vi "Autonomous Independent Backup 4th feb.vi"() -> ()   [LabVIEW 2016]
uses:
  <vilib>/Rock Robotics/WPI/Utilities/WPI_GetSetVariantRefNum.vi
  <vilib>/Rock Robotics/Network Tables/NT Read String.vi
  <vilib>/Rock Robotics/Network Tables/NT Write Numeric Array.vi
  <vilib>/Rock Robotics/WPI/RobotDrive/WPI_RobotDriveArcadeDrive_Standard(NoSaturation).vi
  <vilib>/Rock Robotics/SystemInterfaces/DIO/FPGA_DIOChannel.ctl
  <vilib>/Rock Robotics/WPI/Counter/WPI_CounterDigitalInputToDigitalSource.vi
panel:
  out "Current Movement, for debugging 2":T1 {"Y Joystick Value" scale=1.0..-1.0; "X Joystick Value" scale=-1.0..1.0}
  in  "Array of robot movements 2":T2(array[cluster])=[{"X Joystick Value"=0.39393939393939403, "Y Joystick Value"=0.0, "Delay (sec)"=1.0, "Movement Name"="turn"}, {"X Joystick Value"=-0.3737373737373737, "Y Joystick Value"=0.0, "Delay (sec)"=1.0, "Movement Name"="turn back"}] {"Y Joystick Value" scale=1.0..-1.0; "X Joystick Value" scale=-1.0..1.0}
  out "Encoder Direction 3":string
  out "Encoder Distance 3":dbl
  out "Switch Pressed":bool
  out "Motor Values":dbl[](array[numeric])
  out "Encoder Direction":string
  out "Encoder Distance":dbl
  out "Encoder Direction 2":string
  out "Encoder Distance 2":dbl
  out "Current Movement, for debugging":T1 {"Y Joystick Value" scale=1.0..-1.0; "X Joystick Value" scale=-1.0..1.0}
  in  "Array of robot movements":T2(array[cluster])=[{"X Joystick Value"=0.39393939393939403, "Y Joystick Value"=0.0, "Delay (sec)"=1.0, "Movement Name"="turn"}, {"X Joystick Value"=-0.3737373737373737, "Y Joystick Value"=0.0, "Delay (sec)"=1.0, "Movement Name"="turn back"}] {"Y Joystick Value" scale=1.0..-1.0; "X Joystick Value" scale=-1.0..1.0}
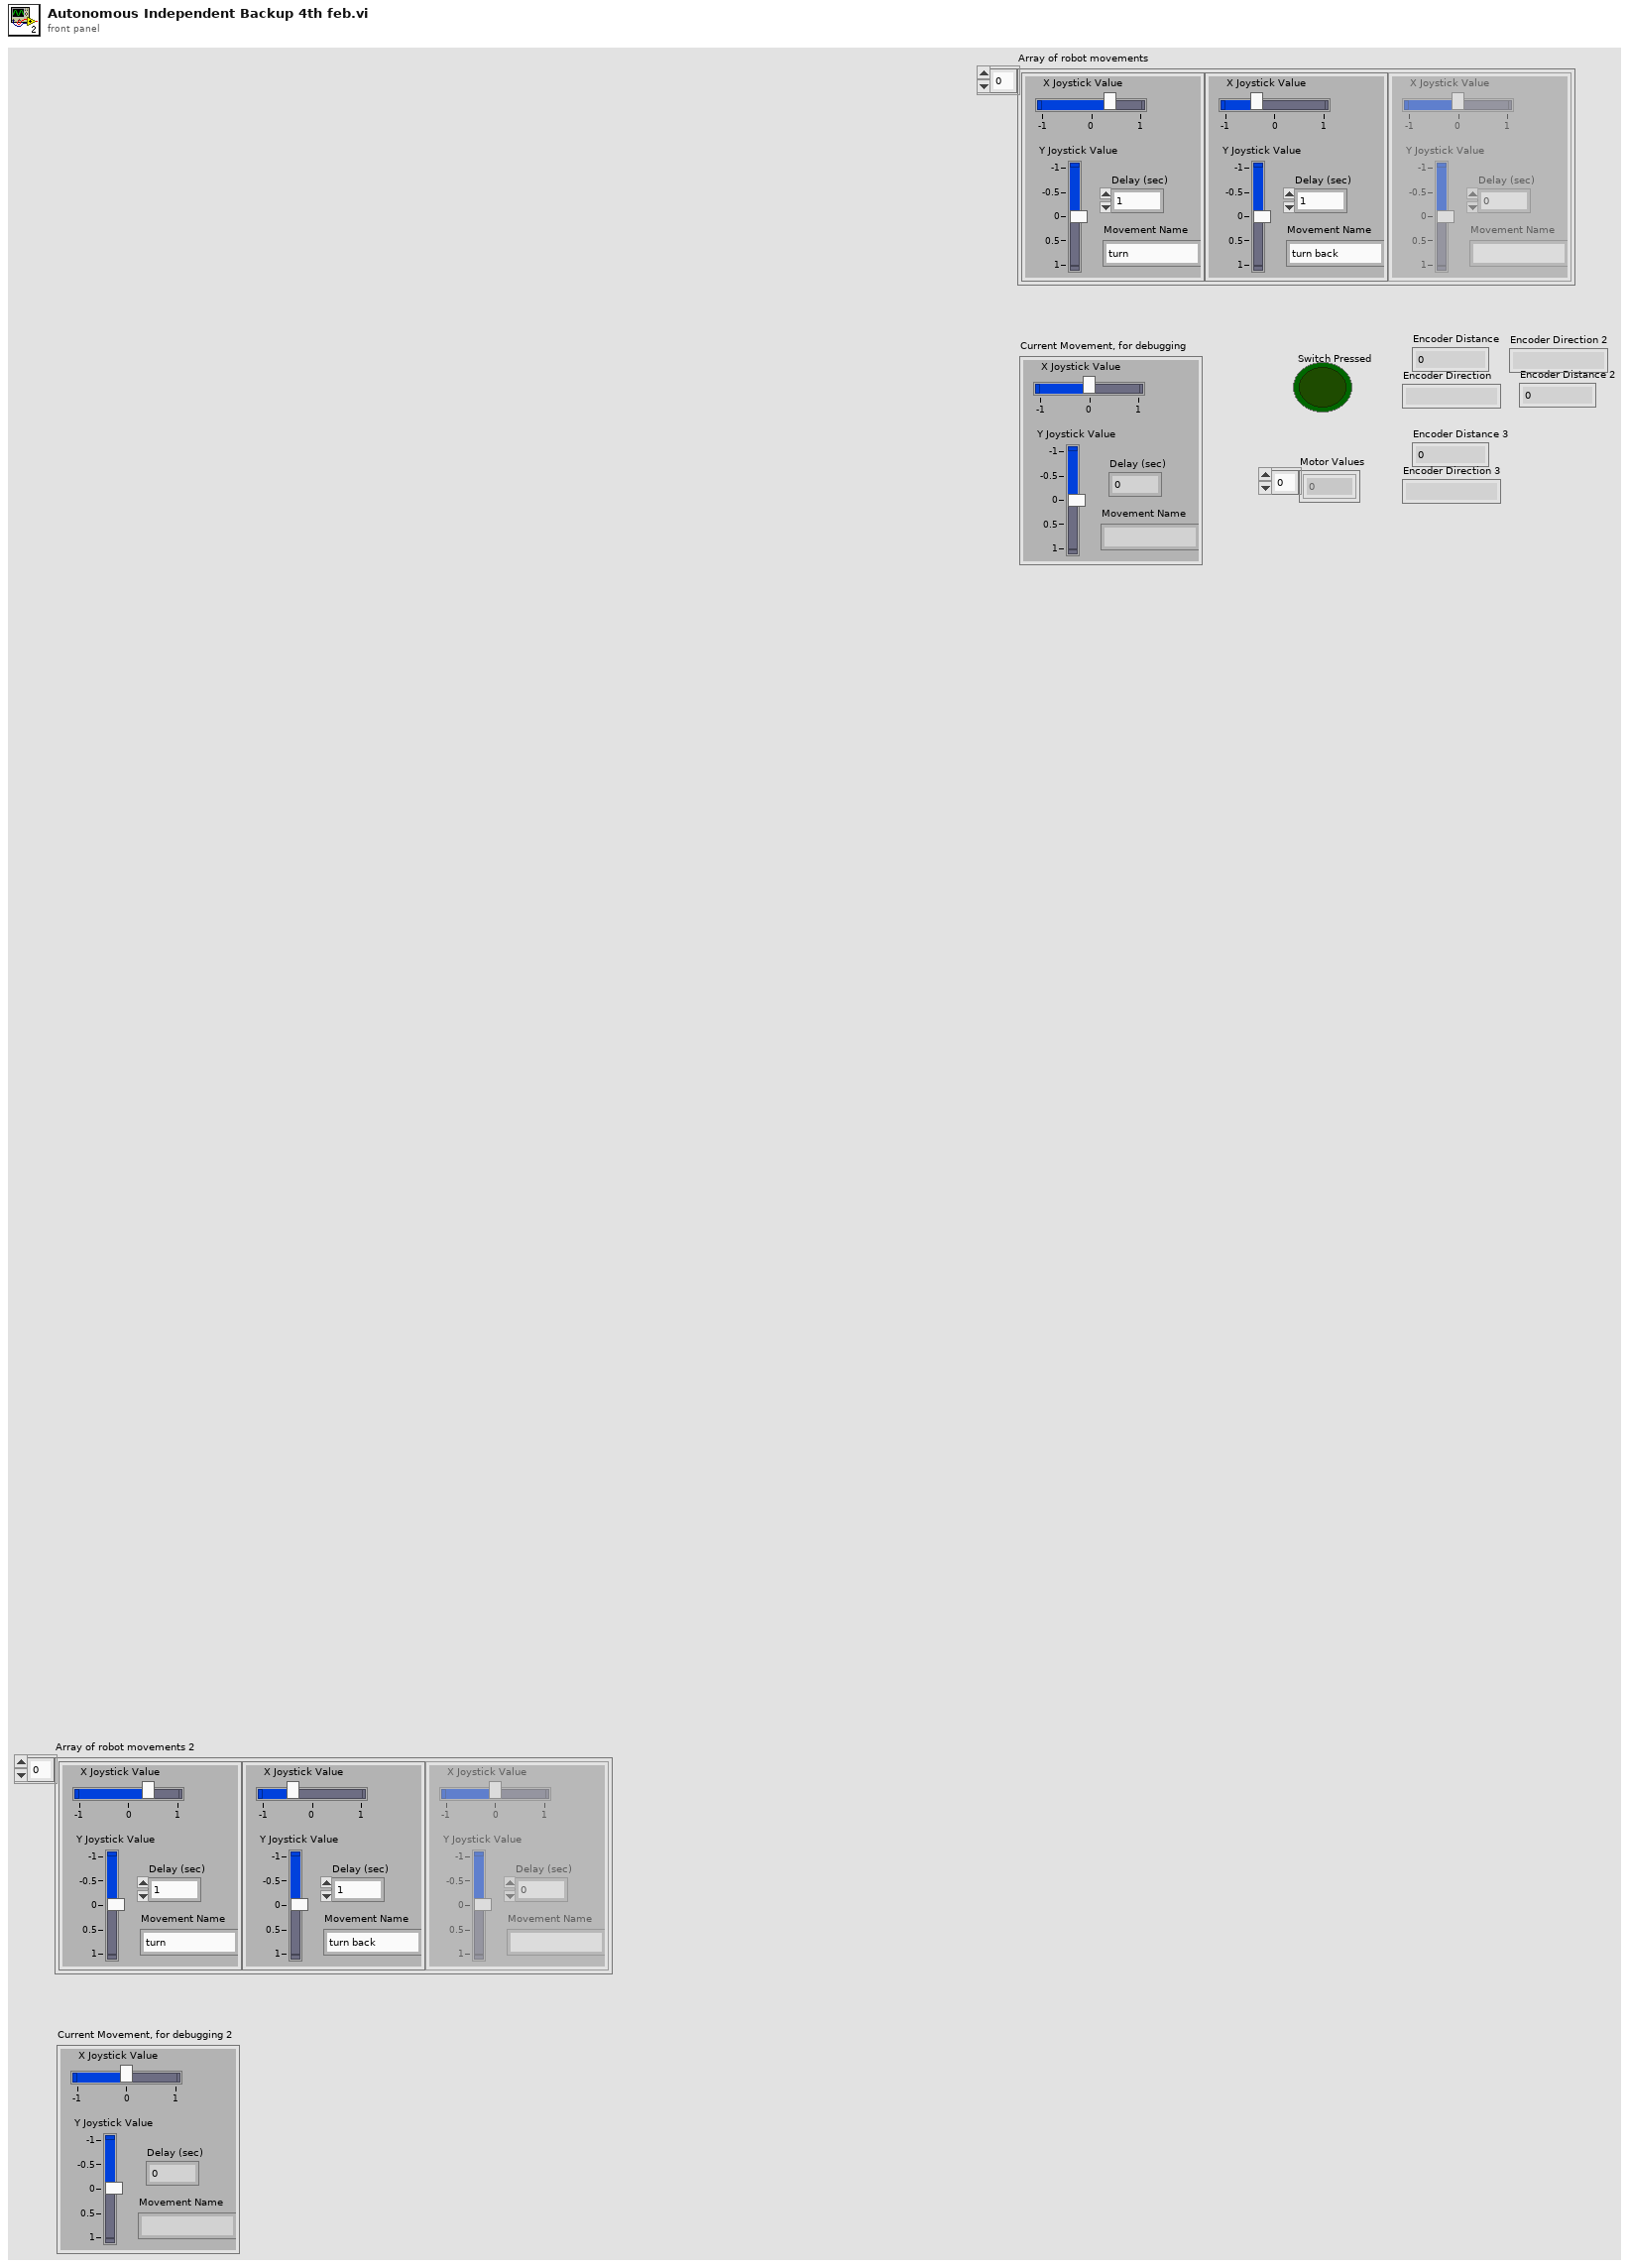
[diagram p1: front panel]
types:
  T1 = cluster{"X Joystick Value":dbl, "Y Joystick Value":dbl, "Delay (sec)":dbl, "Movement Name":string}
  T2 = cluster{"X Joystick Value":dbl, "Y Joystick Value":dbl, "Delay (sec)":dbl, "Movement Name":string}[]
  T3 = typedef "WPI_DriverStationPositionInfo.ctl" = enum16{"1", "2", "3"}
  T4 = typedef "WPI_RobotDriveDevRef.ctl" = cluster{"DevStatus":errorcluster, "Motors[]":T5[], "Square Inputs":bool, "Max Output":dbl}
  T5 = typedef "WPI_MotorControlDeviceRef.ctl" = cluster{"DeviceStatus":errorcluster, "Type":T6, "PWM":cluster{"PWM Channel":T7, "DeadBand":T8}, "CAN":cluster{"Device Number":u8, "SetOutput VI Ref":variant, "GetOutput VI Ref":variant, "Enable VI Ref":variant, "Disable VI Ref":variant, "Data":variant}, "Invert":bool}
  T6 = typedef "WPI_MotorControlType.ctl" = enum16{"PWM", "CAN"}
  T7 = typedef "FPGA_DIOPWMChannel.ctl" = enum8{"PWM 0", "PWM 1", "PWM 2", "PWM 3", "PWM 4", "PWM 5", "PWM 6", "PWM 7", "PWM 8", "PWM 9", "PWM MXP 0", "PWM MXP 1", "PWM MXP 2", "PWM MXP 3", "PWM MXP 4", "PWM MXP 5", "PWM MXP 6", "PWM MXP 7", "PWM MXP 8", "PWM MXP 9", "Invalid"}
  T8 = typedef "WPI_PWMDeadband.ctl" = cluster{"Name":string, "maxPositivePwm":i32, "minPositivePwm":i32, "centerPwm":i32, "maxNegativePwm":i32, "minNegativePwm":i32, "angularRange":u16}
  T9 = typedef "FPGA_DIOChannel.ctl" = enum8{"DIO 0", "DIO 1", "DIO 2", "DIO 3", "DIO 4", "DIO 5", "DIO 6", "DIO 7", "DIO 8", "DIO 9", "DIO MXP 0", "DIO MXP 1", "DIO MXP 2", "DIO MXP 3", "DIO MXP 4", "DIO MXP 5", "DIO MXP 6", "DIO MXP 7", "DIO MXP 8", "DIO MXP 9", "DIO MXP 10", "DIO MXP 11", "DIO MXP 12", "DIO MXP 13", "DIO MXP 14", "DIO MXP 15", "SPI Port CS1", "SPI Port CS2", "SPI Port CS3", "SPI Port MISO", "SPI Port MOSI", "Invalid"}
  T10 = typedef "WPI_DigitalInputDevRef.ctl" = cluster{"DevStatus":errorcluster, "DIO Channel":T9}
  T11 = typedef "FPGA_CounterEncoderSourceConvertionLVSourceType.ctl" = cluster{"DevStatus":errorcluster, "AnalogTriggerMode?":bool, "DigitalMode":cluster{"DIO Channel":T12}, "AnalogTriggerMode":cluster{"AnalogTriggerIndex":T13, "OutputType":T14}}
  T12 = typedef "FPGA_DIODigitalSourceChannel.ctl" = enum8{"DIO 0", "DIO 1", "DIO 2", "DIO 3", "DIO 4", "DIO 5", "DIO 6", "DIO 7", "DIO 8", "DIO 9", "DIO MXP 0", "DIO MXP 1", "DIO MXP 2", "DIO MXP 3", "DIO MXP 4", "DIO MXP 5", "DIO MXP 6", "DIO MXP 7", "DIO MXP 8", "DIO MXP 9", "DIO MXP 10", "DIO MXP 11", "DIO MXP 12", "DIO MXP 13", "DIO MXP 14", "DIO MXP 15", "Disabled"}
  T13 = typedef "FPGA_AnalogTriggerIndex.ctl" = enum8{"Trig 0", "Trig 1", "Trig 2", "Trig 3", "Trig 4", "Trig 5", "Trig 6", "Trig 7", "Invalid"}
  T14 = typedef "FPGA_AnalogTriggerOutType.ctl" = enum16{"InWindow", "TriggerState", "Rising", "Falling"}
  T15 = typedef "WPI_EncoderDevRef.ctl" = cluster{"DevStatus":errorcluster, "EncoderIndex":T16, "CounterIndex":T17, "DistancePerCount":dbl, "Decoding Type":T18}
  T16 = typedef "FPGA_EncoderIdx.ctl" = enum8{"Enc 0", "Enc 1", "Enc 2", "Enc 3", "Enc 4", "Enc 5", "Enc 6", "Enc 7", "Invalid"}
  T17 = typedef "FPGA_CounterCtrSystemIndex.ctl" = enum8{"Ctr 0", "Ctr 1", "Ctr 2", "Ctr 3", "Ctr 4", "Ctr 5", "Ctr 6", "Ctr 7", "Invalid"}
  T18 = typedef "WPI_EncoderType.ctl" = enum16{"1x", "2x", "4x"}
  T19 = typedef "WPI_JoystickDevRef.ctl" = cluster{"Device":T20}
  T20 = typedef "WPI_JoystickDeviceEnum.ctl" = enum16{"USB 0", "USB 1", "USB 2", "USB 3", "USB 4", "USB 5"}
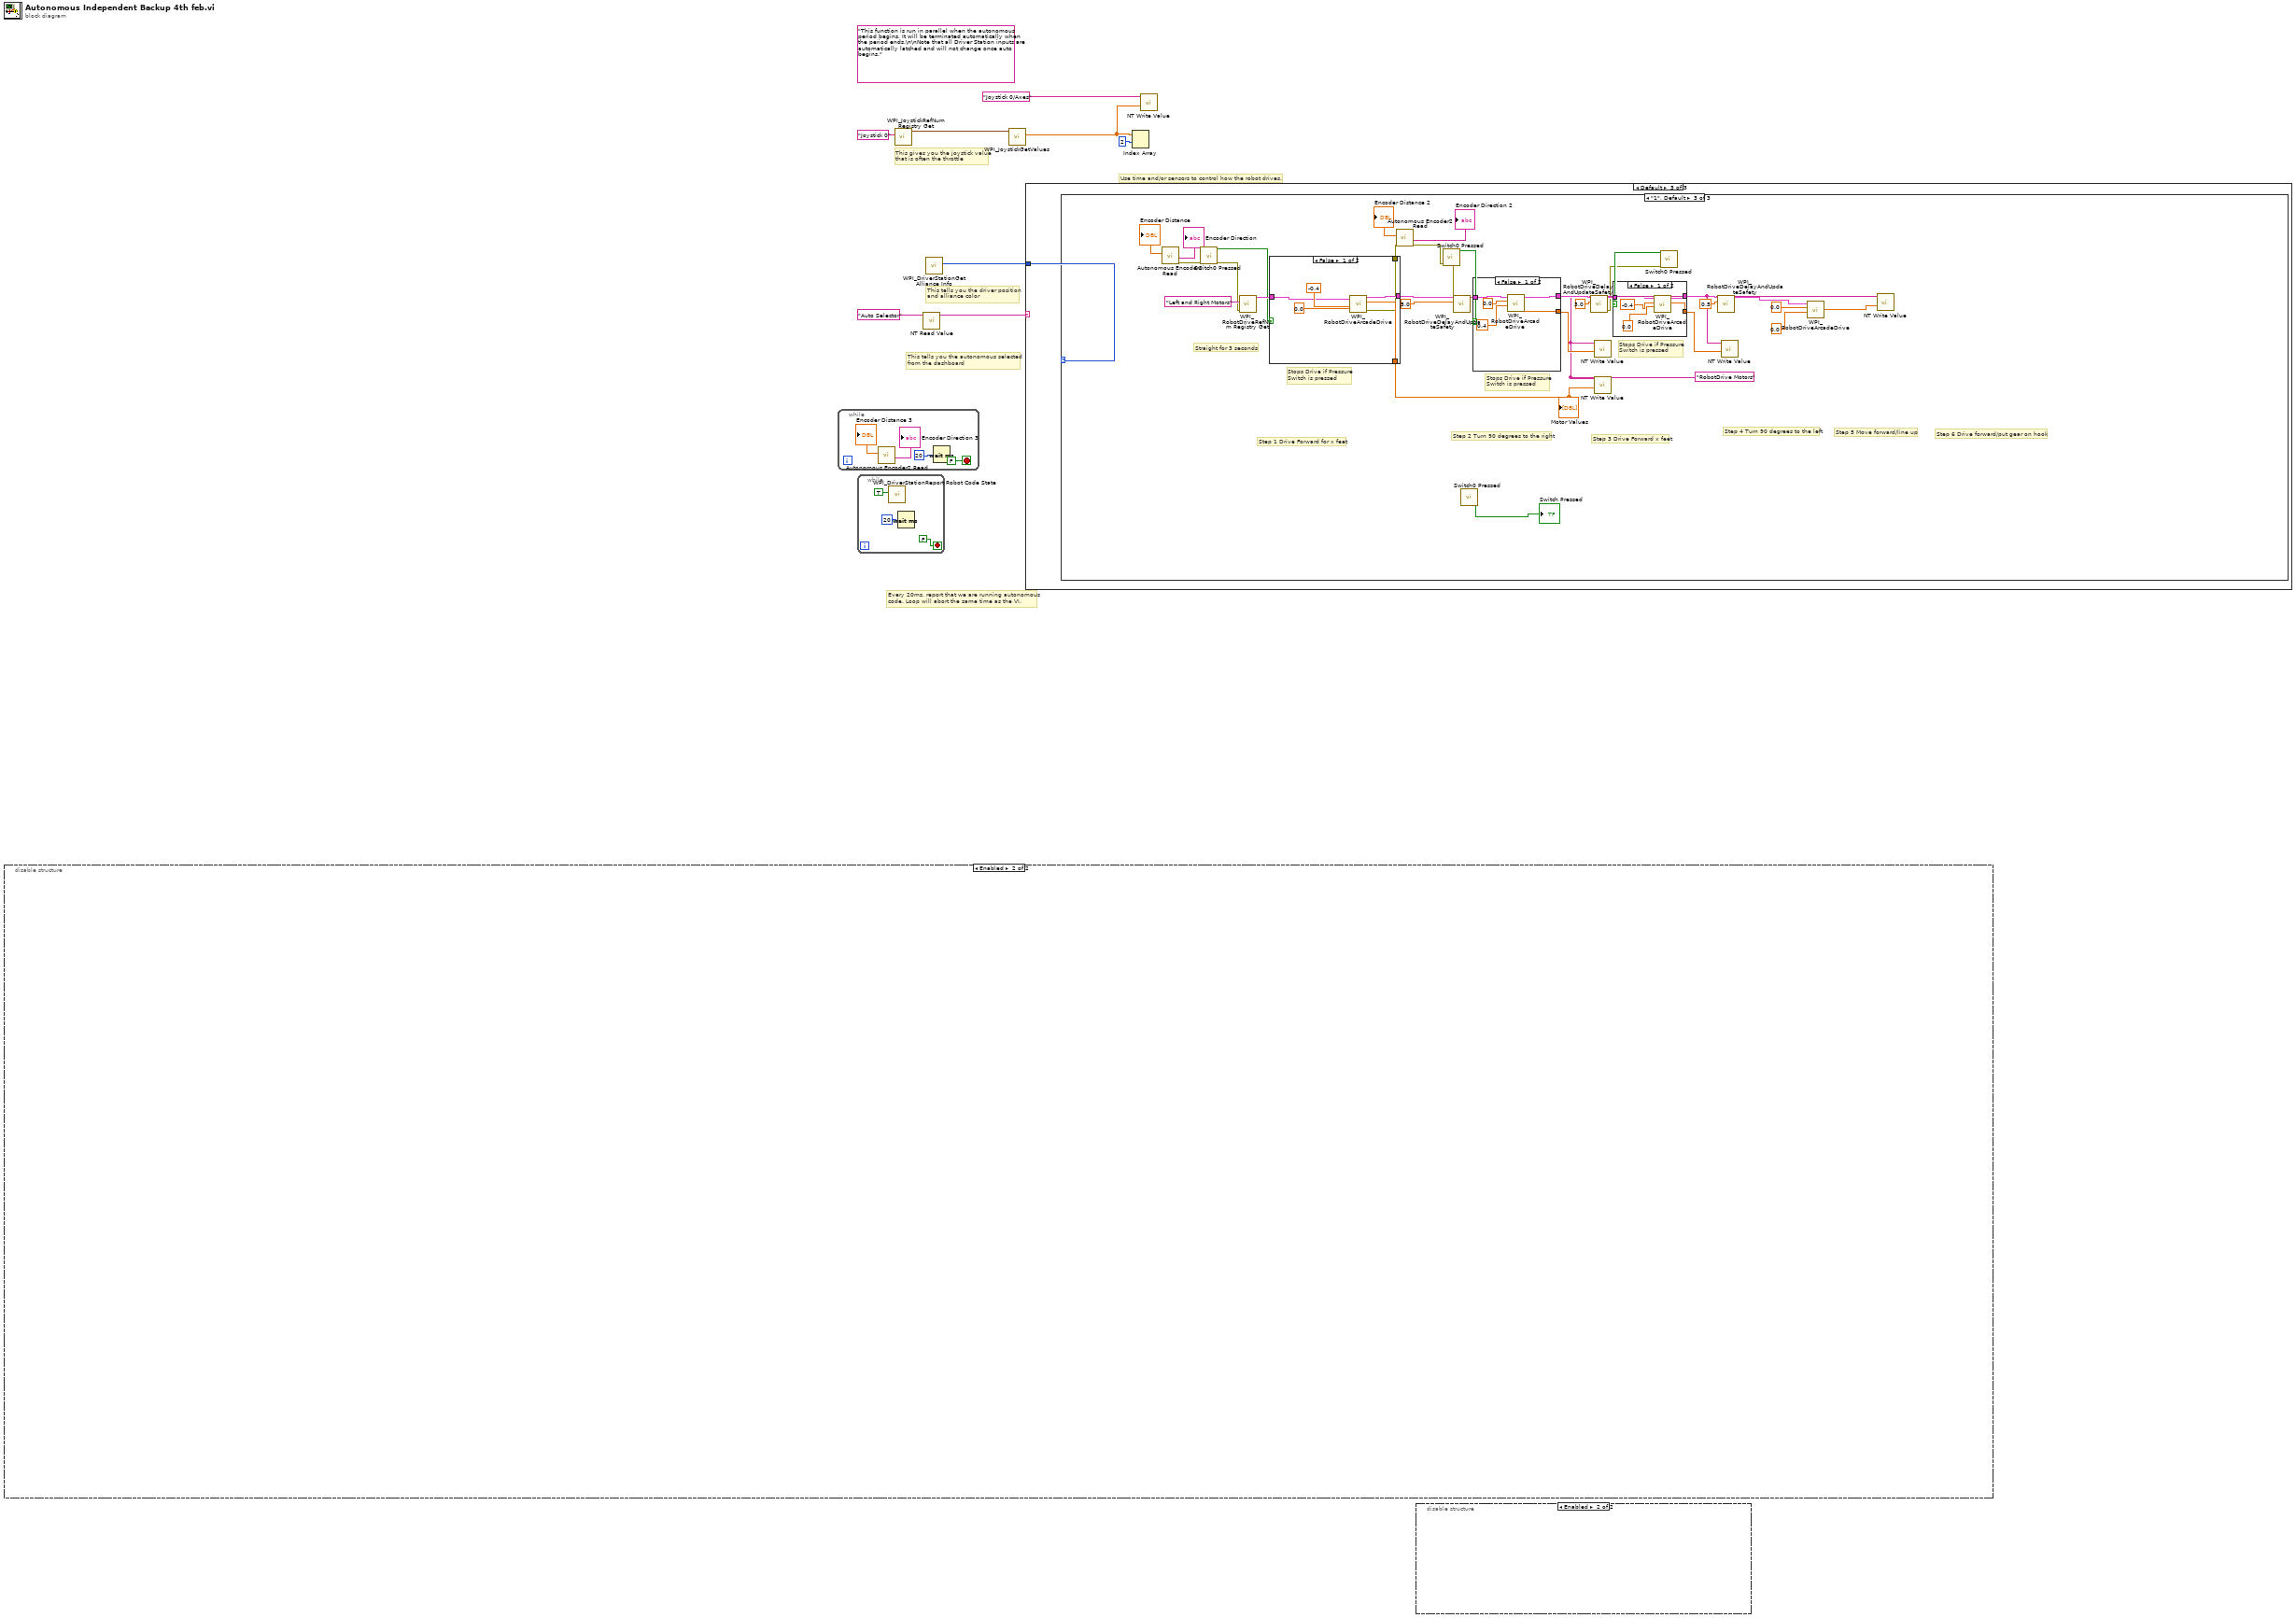
[diagram p0: block diagram]
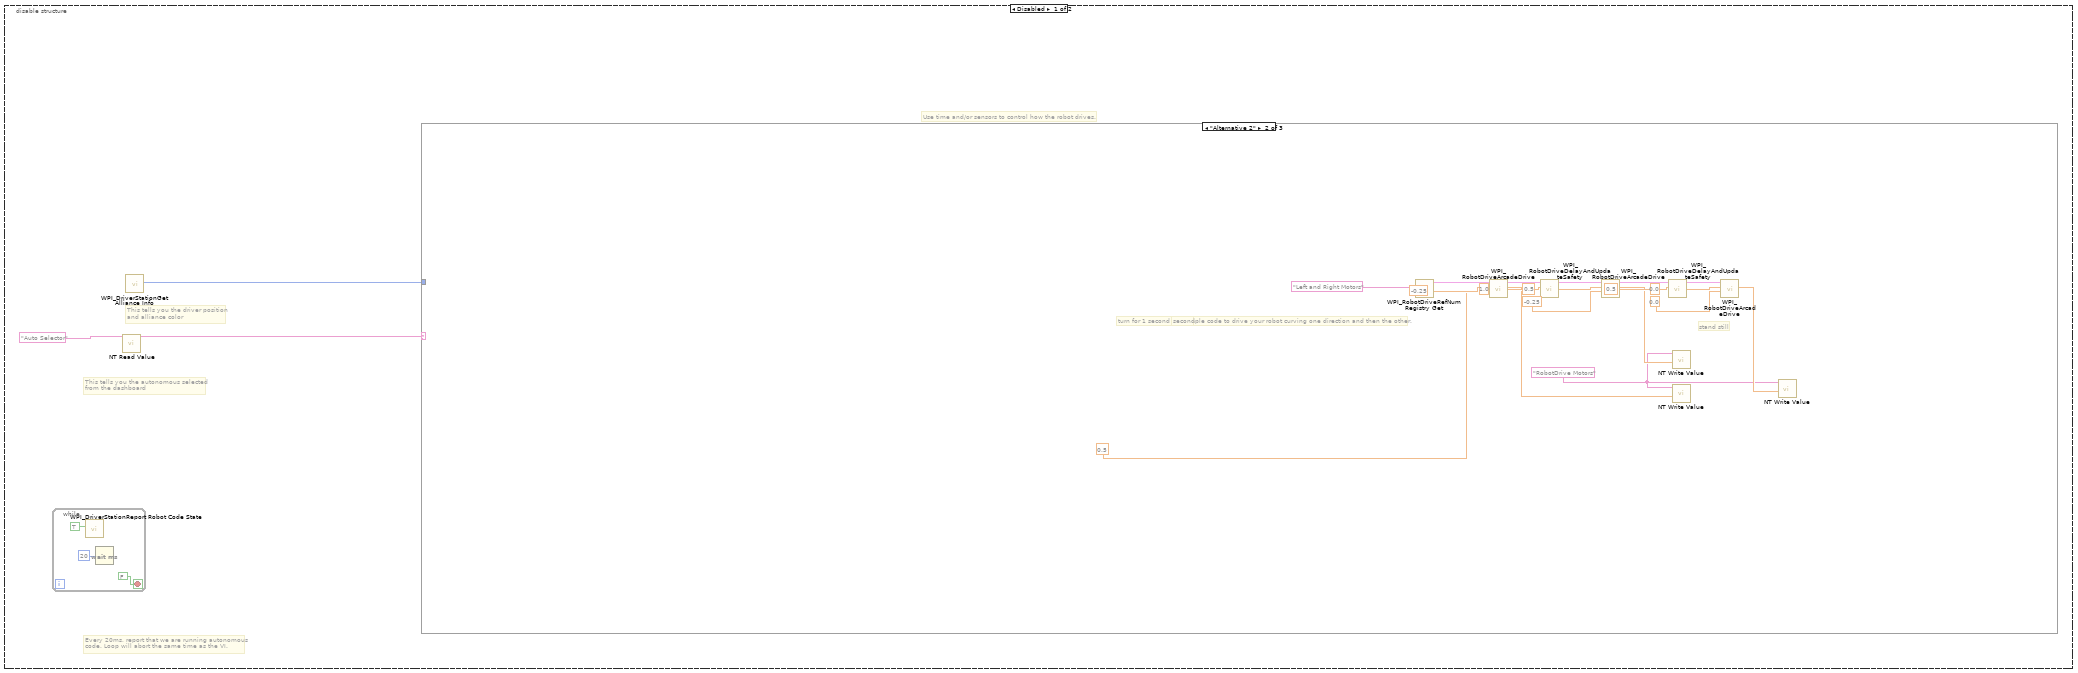
[diagram p2: hidden frame]
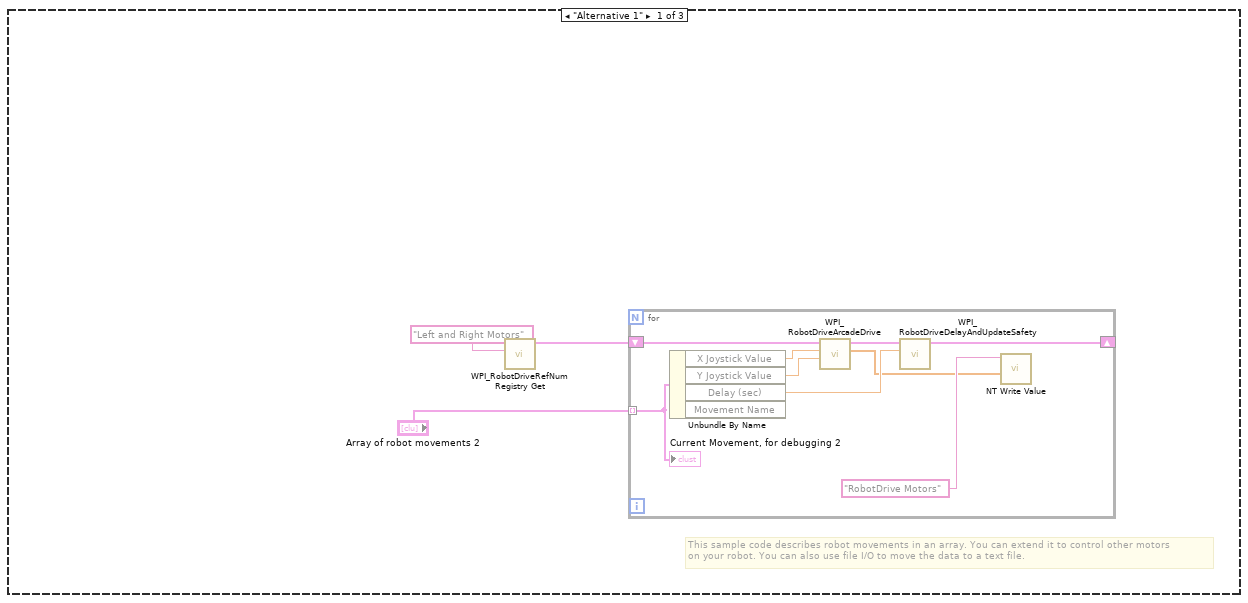
[diagram p3: hidden frame]
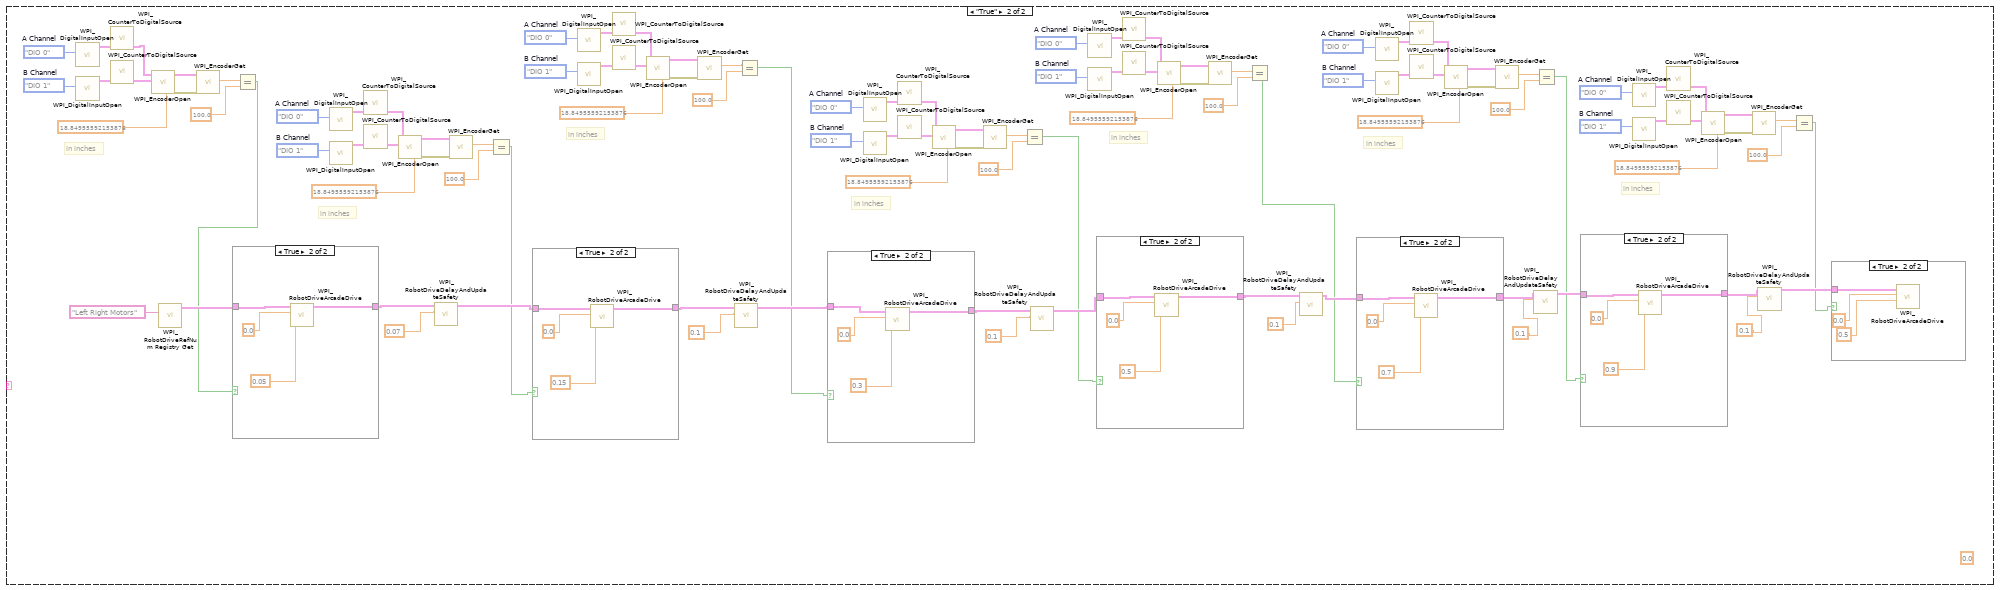
[diagram p5: hidden frame]
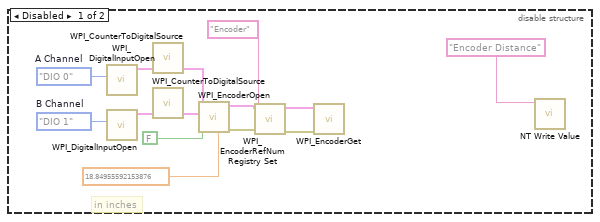
[diagram p13: hidden frame]
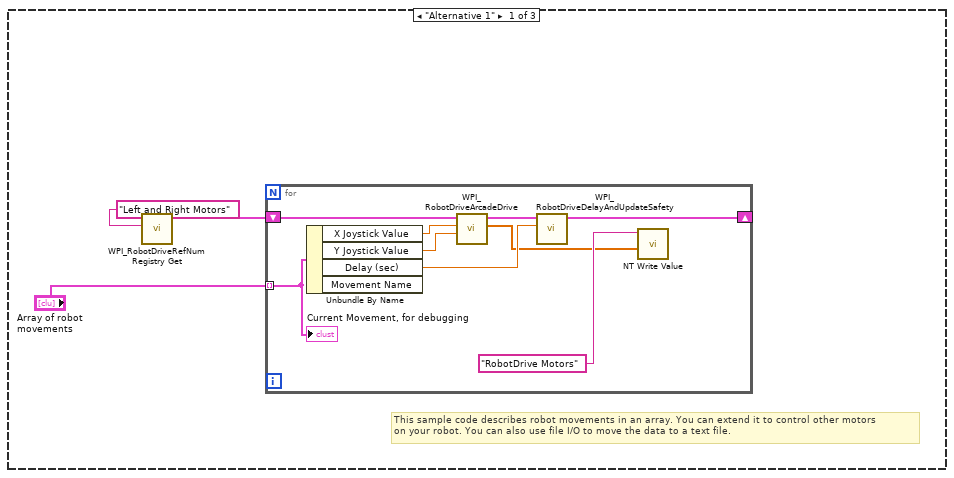
[diagram p14: hidden frame]
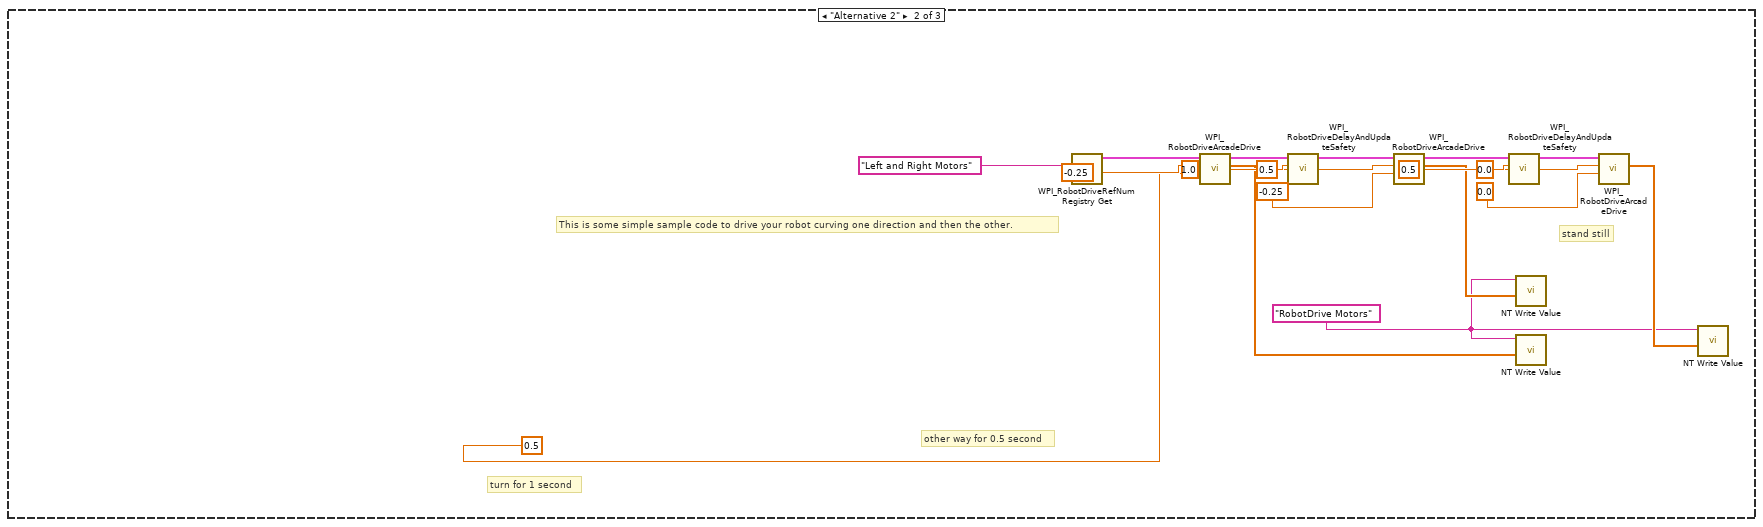
[diagram p15: hidden frame]
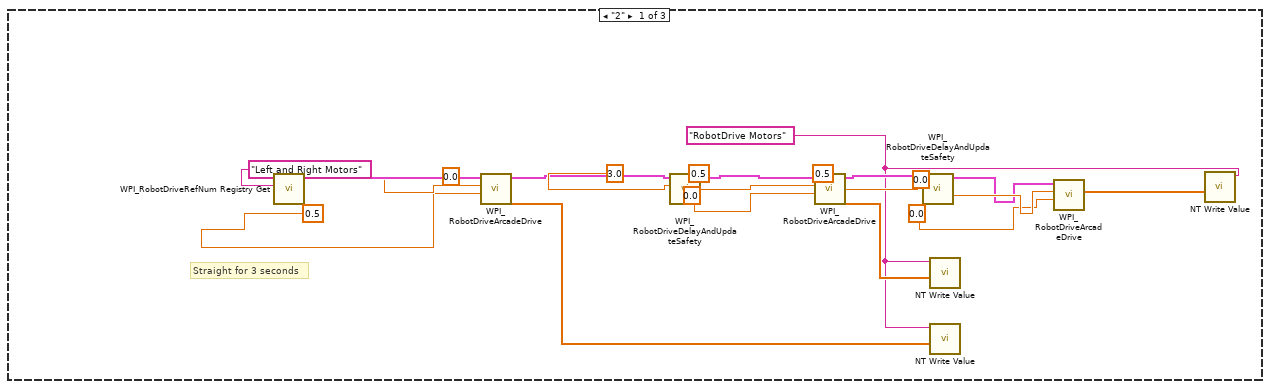
[diagram p16: hidden frame]
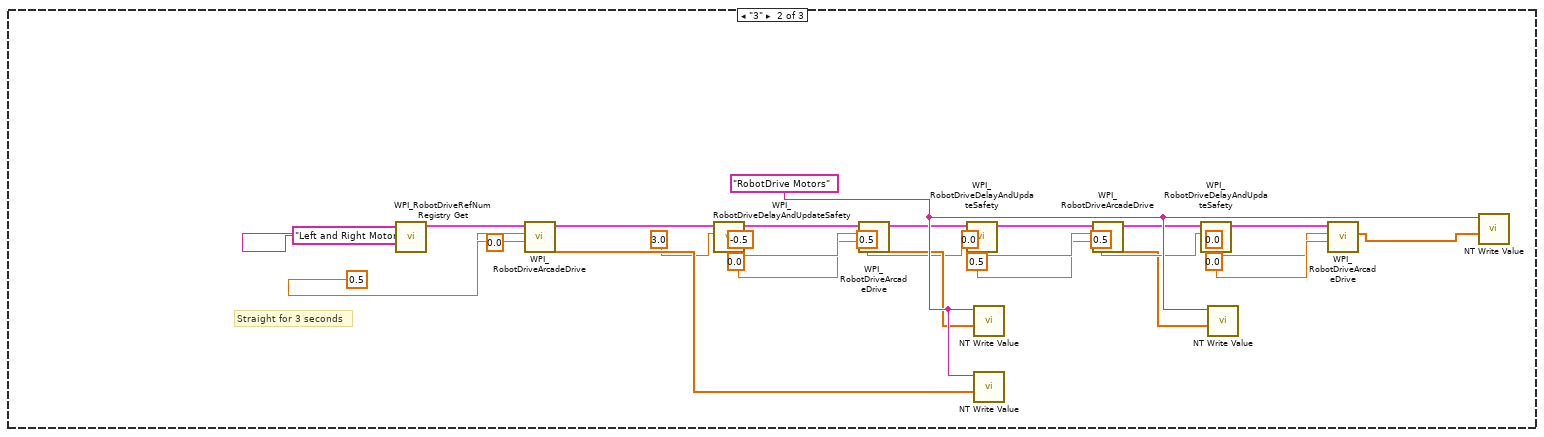
[diagram p17: hidden frame]
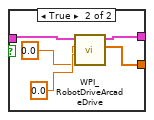
[diagram p18: hidden frame]
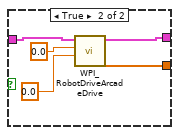
[diagram p19: hidden frame]
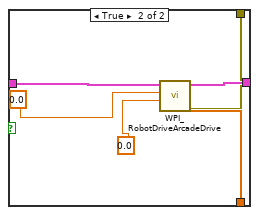
[diagram p20: hidden frame]
diagram:
  (unwired) "This function is run in parallel when the autonomous period begins. It will be terminated automatically when the period ends.\n\nNote that all Driver Station inputs are automatically latched and will not change once auto begins."
  # "This tells you the autonomous selected\nfrom the dashboard"
  # "Every 20ms, report that we are running autonomous\ncode. Loop will abort the same time as the VI."
  # "This gives you the joystick value\nthat is often the throttle"
  # "Use time and/or sensors to control how the robot drives."
  # "This tells you the driver position\nand alliance color"
  n1 = disable-structure shown="Enabled" {
    frame Disabled {
      # "This tells you the autonomous selected\nfrom the dashboard"
      # "Every 20ms, report that we are running autonomous\ncode. Loop will abort the same time as the VI."
      # "Use time and/or sensors to control how the robot drives."
      # "This tells you the driver position\nand alliance color"
      n2 = while {
        stop <- FALSE stop-if-true
        n3 = call <vilib>:"WPI_DriverStationReport Robot Code State.vi"("Autonomous"=TRUE) -> ()  [unwired: 10 in, 1 out]
        n4 = Wait (ms)(milliseconds to wait=u32 20) -> ()  [unwired: 1 out]
      }
      n5 = call-poly <vilib>:"NT Read Value.vi"("Name"="Auto Selector") -> ("String"=w11:string)  [unwired: 9 in, 1 out]
      n6 = call <vilib>:"WPI_DriverStationGet Alliance Info.vi"() -> ("Position"=w10:T3)  [unwired: 11 out]
      n7 = case shown="\"Alternative 2\"" w11 {
        selector: w11 -> [_ _ w42]
        tunnel: w10 -> [_ _ _]
        frame "Alternative 1" {
          # "This sample code describes robot movements in an array. You can extend it to control other motors\non your robot. You can also use file I/O to move the data to a text file."
          n8 = call <vilib>:"WPI_RobotDriveRefNum Registry Get.vi"("refnum name"="Left and Right Motors") -> ("RobotDriveDevRef"=w13:T4)  [unwired: 1 in, 9 out]
          n9 = for {
            shift-right: [w21] -> _
            shift-left: w13 -> [w22]
            tunnel: "Array of robot movements 2" -> [w17] mode=indexing
            n10 = Unbundle By Name(w17) -> ("X Joystick Value"=w20:dbl, "Y Joystick Value"=w19:dbl, "Delay (sec)"=w18:dbl)  [unwired: 1 out]
            n11 = call-poly <vilib>:"WPI_RobotDriveArcadeDrive.vi"("Y axis value"=w19, "X axis value"=w20, "RobotDriveDevRef"=w22) -> ("Motor Values"=w15:dbl[], "RobotDriveDevRef"=w23:T4)  [unwired: 1 in, 6 out]
            n12 = call <vilib>:"WPI_RobotDriveDelayAndUpdateSafety.vi"("Delay (s)"=w18, "RobotDriveDevRef"=w23) -> ("RobotDriveDevRef 2"=w21:T4)  [unwired: 8 in, 1 out]
            n13 = call-poly <vilib>:"NT Write Value.vi"("Numeric Array"=w15, "Name"="RobotDrive Motors") -> ()  [unwired: 9 in, 1 out]
            "Current Movement, for debugging 2" <- w17
          }
        }
        frame "Alternative 2" {
          w25 = "RobotDrive Motors" ("Name")
          # "This is some simple sample code to drive your robot curving one direction and then the other."
          # "stand still"
          # "other way for 0.5 second"
          # "turn for 1 second"
          n14 = call <vilib>:"WPI_RobotDriveRefNum Registry Get.vi"("refnum name"="Left and Right Motors") -> ("RobotDriveDevRef"=w41:T4)  [unwired: 1 in, 9 out]
          n15 = call-poly <vilib>:"WPI_RobotDriveArcadeDrive.vi"("Y axis value"=0.5 ("X axis value"), "X axis value"=-0.25, "RobotDriveDevRef"=w41) -> ("Motor Values"=w24:dbl[], "RobotDriveDevRef"=w34:T4)  [unwired: 1 in, 6 out]
          n16 = call <vilib>:"WPI_RobotDriveDelayAndUpdateSafety.vi"("Delay (s)"=1.0, "RobotDriveDevRef"=w34) -> ("RobotDriveDevRef 2"=w35:T4)  [unwired: 8 in, 1 out]
          n17 = call-poly <vilib>:"WPI_RobotDriveArcadeDrive.vi"("Y axis value"=-0.25 ("X axis value"), "X axis value"=0.5, "RobotDriveDevRef"=w35) -> ("Motor Values"=w26:dbl[], "RobotDriveDevRef"=w36:T4)  [unwired: 1 in, 6 out]
          n18 = call <vilib>:"WPI_RobotDriveDelayAndUpdateSafety.vi"("Delay (s)"=0.5, "RobotDriveDevRef"=w36) -> ("RobotDriveDevRef 2"=w37:T4)  [unwired: 8 in, 1 out]
          n19 = call-poly <vilib>:"NT Write Value.vi"("Numeric Array"=w26, "Name"=w25) -> ()  [unwired: 9 in, 1 out]
          n20 = call-poly <vilib>:"NT Write Value.vi"("Numeric Array"=w24, "Name"=w25) -> ()  [unwired: 9 in, 1 out]
          n21 = call-poly <vilib>:"WPI_RobotDriveArcadeDrive.vi"("Y axis value"=0.0 ("X axis value"), "X axis value"=0.0, "RobotDriveDevRef"=w37) -> ("Motor Values"=w27:dbl[])  [unwired: 1 in, 7 out]
          n22 = call-poly <vilib>:"NT Write Value.vi"("Numeric Array"=w27, "Name"=w25) -> ()  [unwired: 9 in, 1 out]
        }
        frame Default {
          n23 = case shown="\"False\", Default" w42 {
            frame "False", Default {
            }
            frame "True" {
              w55 = FPGA_DIOChannel."DIO 1"  # B Channel
              w54 = FPGA_DIOChannel."DIO 0"  # A Channel
              w68 = FPGA_DIOChannel."DIO 1"  # B Channel
              w67 = FPGA_DIOChannel."DIO 0"  # A Channel
              w79 = FPGA_DIOChannel."DIO 1"  # B Channel
              w78 = FPGA_DIOChannel."DIO 0"  # A Channel
              w91 = FPGA_DIOChannel."DIO 1"  # B Channel
              w90 = FPGA_DIOChannel."DIO 0"  # A Channel
              w103 = FPGA_DIOChannel."DIO 1"  # B Channel
              w102 = FPGA_DIOChannel."DIO 0"  # A Channel
              w115 = FPGA_DIOChannel."DIO 1"  # B Channel
              w114 = FPGA_DIOChannel."DIO 0"  # A Channel
              w126 = FPGA_DIOChannel."DIO 1"  # B Channel
              w125 = FPGA_DIOChannel."DIO 0"  # A Channel
              (unwired) 0.0 ("Distance")
              # "in inches"
              # "in inches"
              # "in inches"
              # "in inches"
              # "in inches"
              # "in inches"
              # "in inches"
              n24 = call <vilib>:"WPI_DigitalInputOpen.vi"("DIO Channel"=w125) -> ("DigitalInputDevRef"=w122:T10)  [unwired: 1 in, 9 out]
              n25 = call <vilib>:"WPI_DigitalInputOpen.vi"("DIO Channel"=w126) -> ("DigitalInputDevRef"=w123:T10)  [unwired: 1 in, 9 out]
              n26 = call-poly <vilib>:"WPI_CounterToDigitalSource.vi"("DigitalInputDevRef"=w122) -> ("Digital Source"=w43:T11)  [unwired: 6 out]
              n27 = call-poly <vilib>:"WPI_CounterToDigitalSource.vi"("DigitalInputDevRef"=w123) -> ("Digital Source"=w124:T11)  [unwired: 6 out]
              n28 = call <vilib>:"WPI_EncoderOpen.vi"("DistancePerCount"=18.84955592153876, "BSource"=w124, "ASource"=w43) -> ("error out"=w119:errorcluster, "EncoderDevRef"=w120:T15)  [unwired: 5 in, 2 out]
              n29 = call <vilib>:"WPI_RobotDriveRefNum Registry Get.vi"("refnum name"="Left Right Motors") -> ("RobotDriveDevRef"=w145:T4)  [unwired: 9 in, 1 out]
              n30 = call <vilib>:"WPI_EncoderGet.vi"("error in (no error)"=w119, "EncoderDevRef"=w120) -> ("Distance"=w118:dbl)  [unwired: 4 in, 5 out]
              n31 = Equal?(x=w118, y=100.0) -> (x = y?=w116:bool)
              n32 = case shown="True" w116 {
                tunnel: w145 -> [w175 w179]
                tunnel: [w175 w176] -> w144
                frame False {
                }
                frame True {
                  n33 = call-poly <vilib>:"WPI_RobotDriveArcadeDrive.vi"("Y axis value"=0.05, "X axis value"=0.0, "RobotDriveDevRef"=w179) -> ("RobotDriveDevRef"=w176:T4)  [unwired: 6 in, 2 out]
                }
              }
              n34 = call <vilib>:"WPI_DigitalInputOpen.vi"("DIO Channel"=w114) -> ("DigitalInputDevRef"=w111:T10)  [unwired: 1 in, 9 out]
              n35 = call <vilib>:"WPI_DigitalInputOpen.vi"("DIO Channel"=w115) -> ("DigitalInputDevRef"=w112:T10)  [unwired: 1 in, 9 out]
              n36 = call-poly <vilib>:"WPI_CounterToDigitalSource.vi"("DigitalInputDevRef"=w111) -> ("Digital Source"=w110:T11)  [unwired: 6 out]
              n37 = call-poly <vilib>:"WPI_CounterToDigitalSource.vi"("DigitalInputDevRef"=w112) -> ("Digital Source"=w113:T11)  [unwired: 6 out]
              n38 = call <vilib>:"WPI_EncoderOpen.vi"("DistancePerCount"=18.84955592153876, "BSource"=w113, "ASource"=w110) -> ("error out"=w107:errorcluster, "EncoderDevRef"=w108:T15)  [unwired: 5 in, 2 out]
              n39 = call <vilib>:"WPI_RobotDriveDelayAndUpdateSafety.vi"("Delay (s)"=0.07, "RobotDriveDevRef"=w144) -> ("RobotDriveDevRef 2"=w140:T4)  [unwired: 8 in, 1 out]
              n40 = call <vilib>:"WPI_EncoderGet.vi"("error in (no error)"=w107, "EncoderDevRef"=w108) -> ("Distance"=w106:dbl)  [unwired: 4 in, 5 out]
              n41 = Equal?(x=w106, y=100.0) -> (x = y?=w104:bool)
              n42 = case shown="True" w104 {
                tunnel: w140 -> [w170 w174]
                tunnel: [w170 w171] -> w142
                frame False {
                }
                frame True {
                  n43 = call-poly <vilib>:"WPI_RobotDriveArcadeDrive.vi"("Y axis value"=0.15, "X axis value"=0.0, "RobotDriveDevRef"=w174) -> ("RobotDriveDevRef"=w171:T4)  [unwired: 6 in, 2 out]
                }
              }
              n44 = call <vilib>:"WPI_DigitalInputOpen.vi"("DIO Channel"=w102) -> ("DigitalInputDevRef"=w99:T10)  [unwired: 1 in, 9 out]
              n45 = call <vilib>:"WPI_DigitalInputOpen.vi"("DIO Channel"=w103) -> ("DigitalInputDevRef"=w100:T10)  [unwired: 1 in, 9 out]
              n46 = call-poly <vilib>:"WPI_CounterToDigitalSource.vi"("DigitalInputDevRef"=w99) -> ("Digital Source"=w98:T11)  [unwired: 6 out]
              n47 = call-poly <vilib>:"WPI_CounterToDigitalSource.vi"("DigitalInputDevRef"=w100) -> ("Digital Source"=w101:T11)  [unwired: 6 out]
              n48 = call <vilib>:"WPI_EncoderOpen.vi"("DistancePerCount"=18.84955592153876, "BSource"=w101, "ASource"=w98) -> ("error out"=w95:errorcluster, "EncoderDevRef"=w96:T15)  [unwired: 5 in, 2 out]
              n49 = call <vilib>:"WPI_EncoderGet.vi"("error in (no error)"=w95, "EncoderDevRef"=w96) -> ("Distance"=w94:dbl)  [unwired: 4 in, 5 out]
              n50 = call <vilib>:"WPI_RobotDriveDelayAndUpdateSafety.vi"("Delay (s)"=0.1, "RobotDriveDevRef"=w142) -> ("RobotDriveDevRef 2"=w137:T4)  [unwired: 8 in, 1 out]
              n51 = Equal?(x=w94, y=100.0) -> (x = y?=w92:bool)
              n52 = case shown="True" w92 {
                tunnel: w137 -> [w165 w169]
                tunnel: [w165 w166] -> w139
                frame False {
                }
                frame True {
                  n53 = call-poly <vilib>:"WPI_RobotDriveArcadeDrive.vi"("Y axis value"=0.3, "X axis value"=0.0, "RobotDriveDevRef"=w169) -> ("RobotDriveDevRef"=w166:T4)  [unwired: 6 in, 2 out]
                }
              }
              n54 = call <vilib>:"WPI_DigitalInputOpen.vi"("DIO Channel"=w90) -> ("DigitalInputDevRef"=w87:T10)  [unwired: 1 in, 9 out]
              n55 = call <vilib>:"WPI_DigitalInputOpen.vi"("DIO Channel"=w91) -> ("DigitalInputDevRef"=w88:T10)  [unwired: 1 in, 9 out]
              n56 = call-poly <vilib>:"WPI_CounterToDigitalSource.vi"("DigitalInputDevRef"=w87) -> ("Digital Source"=w86:T11)  [unwired: 6 out]
              n57 = call-poly <vilib>:"WPI_CounterToDigitalSource.vi"("DigitalInputDevRef"=w88) -> ("Digital Source"=w89:T11)  [unwired: 6 out]
              n58 = call <vilib>:"WPI_EncoderOpen.vi"("DistancePerCount"=18.84955592153876, "BSource"=w89, "ASource"=w86) -> ("error out"=w83:errorcluster, "EncoderDevRef"=w84:T15)  [unwired: 5 in, 2 out]
              n59 = call <vilib>:"WPI_EncoderGet.vi"("error in (no error)"=w83, "EncoderDevRef"=w84) -> ("Distance"=w82:dbl)  [unwired: 4 in, 5 out]
              n60 = Equal?(x=w82, y=100.0) -> (x = y?=w80:bool)
              n61 = call <vilib>:"WPI_RobotDriveDelayAndUpdateSafety.vi"("Delay (s)"=0.1, "RobotDriveDevRef"=w139) -> ("RobotDriveDevRef 2"=w135:T4)  [unwired: 8 in, 1 out]
              n62 = call <vilib>:"WPI_DigitalInputOpen.vi"("DIO Channel"=w78) -> ("DigitalInputDevRef"=w75:T10)  [unwired: 1 in, 9 out]
              n63 = call <vilib>:"WPI_DigitalInputOpen.vi"("DIO Channel"=w79) -> ("DigitalInputDevRef"=w76:T10)  [unwired: 1 in, 9 out]
              n64 = case shown="True" w80 {
                tunnel: w135 -> [w160 w164]
                tunnel: [w160 w161] -> w136
                frame False {
                }
                frame True {
                  n65 = call-poly <vilib>:"WPI_RobotDriveArcadeDrive.vi"("Y axis value"=0.5, "X axis value"=0.0, "RobotDriveDevRef"=w164) -> ("RobotDriveDevRef"=w161:T4)  [unwired: 6 in, 2 out]
                }
              }
              n66 = call-poly <vilib>:"WPI_CounterToDigitalSource.vi"("DigitalInputDevRef"=w75) -> ("Digital Source"=w74:T11)  [unwired: 6 out]
              n67 = call-poly <vilib>:"WPI_CounterToDigitalSource.vi"("DigitalInputDevRef"=w76) -> ("Digital Source"=w77:T11)  [unwired: 6 out]
              n68 = call <vilib>:"WPI_EncoderOpen.vi"("DistancePerCount"=18.84955592153876, "BSource"=w77, "ASource"=w74) -> ("error out"=w71:errorcluster, "EncoderDevRef"=w72:T15)  [unwired: 5 in, 2 out]
              n69 = call <vilib>:"WPI_EncoderGet.vi"("error in (no error)"=w71, "EncoderDevRef"=w72) -> ("Distance"=w70:dbl)  [unwired: 4 in, 5 out]
              n70 = Equal?(x=w70, y=100.0) -> (x = y?=w57:bool)
              n71 = call <vilib>:"WPI_RobotDriveDelayAndUpdateSafety.vi"("Delay (s)"=0.1, "RobotDriveDevRef"=w136) -> ("RobotDriveDevRef 2"=w131:T4)  [unwired: 8 in, 1 out]
              n72 = case shown="True" w57 {
                tunnel: w131 -> [w155 w159]
                tunnel: [w155 w156] -> w132
                frame False {
                }
                frame True {
                  n73 = call-poly <vilib>:"WPI_RobotDriveArcadeDrive.vi"("Y axis value"=0.7, "X axis value"=0.0, "RobotDriveDevRef"=w159) -> ("RobotDriveDevRef"=w156:T4)  [unwired: 6 in, 2 out]
                }
              }
              n74 = call <vilib>:"WPI_DigitalInputOpen.vi"("DIO Channel"=w67) -> ("DigitalInputDevRef"=w64:T10)  [unwired: 1 in, 9 out]
              n75 = call <vilib>:"WPI_DigitalInputOpen.vi"("DIO Channel"=w68) -> ("DigitalInputDevRef"=w65:T10)  [unwired: 1 in, 9 out]
              n76 = call-poly <vilib>:"WPI_CounterToDigitalSource.vi"("DigitalInputDevRef"=w64) -> ("Digital Source"=w63:T11)  [unwired: 6 out]
              n77 = call-poly <vilib>:"WPI_CounterToDigitalSource.vi"("DigitalInputDevRef"=w65) -> ("Digital Source"=w66:T11)  [unwired: 6 out]
              n78 = call <vilib>:"WPI_EncoderOpen.vi"("DistancePerCount"=18.84955592153876, "BSource"=w66, "ASource"=w63) -> ("error out"=w60:errorcluster, "EncoderDevRef"=w61:T15)  [unwired: 5 in, 2 out]
              n79 = call <vilib>:"WPI_EncoderGet.vi"("error in (no error)"=w60, "EncoderDevRef"=w61) -> ("Distance"=w59:dbl)  [unwired: 4 in, 5 out]
              n80 = call <vilib>:"WPI_RobotDriveDelayAndUpdateSafety.vi"("Delay (s)"=0.1, "RobotDriveDevRef"=w132) -> ("RobotDriveDevRef 2"=w128:T4)  [unwired: 8 in, 1 out]
              n81 = Equal?(x=w59, y=100.0) -> (x = y?=w56:bool)
              n82 = case shown="True" w56 {
                tunnel: w128 -> [w150 w154]
                tunnel: [w150 w151] -> w129
                frame False {
                }
                frame True {
                  n83 = call-poly <vilib>:"WPI_RobotDriveArcadeDrive.vi"("Y axis value"=0.9, "X axis value"=0.0, "RobotDriveDevRef"=w154) -> ("RobotDriveDevRef"=w151:T4)  [unwired: 6 in, 2 out]
                }
              }
              n84 = call <vilib>:"WPI_DigitalInputOpen.vi"("DIO Channel"=w54) -> ("DigitalInputDevRef"=w51:T10)  [unwired: 1 in, 9 out]
              n85 = call <vilib>:"WPI_DigitalInputOpen.vi"("DIO Channel"=w55) -> ("DigitalInputDevRef"=w52:T10)  [unwired: 1 in, 9 out]
              n86 = call-poly <vilib>:"WPI_CounterToDigitalSource.vi"("DigitalInputDevRef"=w51) -> ("Digital Source"=w50:T11)  [unwired: 6 out]
              n87 = call-poly <vilib>:"WPI_CounterToDigitalSource.vi"("DigitalInputDevRef"=w52) -> ("Digital Source"=w53:T11)  [unwired: 6 out]
              n88 = call <vilib>:"WPI_EncoderOpen.vi"("DistancePerCount"=18.84955592153876, "BSource"=w53, "ASource"=w50) -> ("error out"=w47:errorcluster, "EncoderDevRef"=w48:T15)  [unwired: 5 in, 2 out]
              n89 = call <vilib>:"WPI_EncoderGet.vi"("error in (no error)"=w47, "EncoderDevRef"=w48) -> ("Distance"=w46:dbl)  [unwired: 4 in, 5 out]
              n90 = call <vilib>:"WPI_RobotDriveDelayAndUpdateSafety.vi"("Delay (s)"=0.1, "RobotDriveDevRef"=w129) -> ("RobotDriveDevRef 2"=w127:T4)  [unwired: 8 in, 1 out]
              n91 = Equal?(x=w46, y=100.0) -> (x = y?=w44:bool)
              n92 = case shown="True" w44 {
                tunnel: w127 -> [_ w149]
                frame False {
                }
                frame True {
                  n93 = call-poly <vilib>:"WPI_RobotDriveArcadeDrive.vi"("Y axis value"=0.5, "X axis value"=0.0, "RobotDriveDevRef"=w149) -> ()  [unwired: 6 in, 3 out]
                }
              }
            }
          }
        }
      }
    }
    frame Enabled {
    }
  }
  n94 = while {
    stop <- FALSE stop-if-true
    n95 = call "Autonomous Encoder2 Read.vi"() -> ("Encoder Direction"=→"Encoder Direction 3":string, "Encoder Distance"=→"Encoder Distance 3":dbl)  [unwired: 9 in, 1 out]
    n96 = Wait (ms)(milliseconds to wait=u32 20) -> ()  [unwired: 1 out]
  }
  n97 = while {
    stop <- FALSE stop-if-true
    n98 = call <vilib>:"WPI_DriverStationReport Robot Code State.vi"("Autonomous"=TRUE) -> ()  [unwired: 10 in, 1 out]
    n99 = Wait (ms)(milliseconds to wait=u32 20) -> ()  [unwired: 1 out]
  }
  n100 = call <vilib>:"WPI_JoystickRefNum Registry Get.vi"("refnum name"="Joystick 0") -> ("JoystickDevRef"=w7:T19)  [unwired: 1 in, 9 out]
  n101 = call-poly <vilib>:"NT Read Value.vi"("Name"="Auto Selector") -> ("String"=w4:string)  [unwired: 9 in, 1 out]
  n102 = call <vilib>:"WPI_DriverStationGet Alliance Info.vi"() -> ("Position"=w1:T3)  [unwired: 11 out]
  n103 = call <vilib>:"WPI_JoystickGetValues.vi"("JoystickDevRef"=w7) -> ("Axes"=w3:dbl[])  [unwired: 6 in, 4 out]
  n104 = case shown="Default" w4 {
    tunnel: w1 -> [_ _ w220]
    frame "Alternative 1" {
      # "This sample code describes robot movements in an array. You can extend it to control other motors\non your robot. You can also use file I/O to move the data to a text file."
      n105 = call <vilib>:"WPI_RobotDriveRefNum Registry Get.vi"("refnum name"="Left and Right Motors") -> ("RobotDriveDevRef"=w191:T4)  [unwired: 1 in, 9 out]
      n106 = for {
        shift-right: [w199] -> _
        shift-left: w191 -> [w200]
        tunnel: "Array of robot movements" -> [w195] mode=indexing
        n107 = Unbundle By Name(w195) -> ("X Joystick Value"=w198:dbl, "Y Joystick Value"=w197:dbl, "Delay (sec)"=w196:dbl)  [unwired: 1 out]
        n108 = call-poly <vilib>:"WPI_RobotDriveArcadeDrive.vi"("Y axis value"=w197, "X axis value"=w198, "RobotDriveDevRef"=w200) -> ("Motor Values"=w193:dbl[], "RobotDriveDevRef"=w201:T4)  [unwired: 1 in, 6 out]
        n109 = call <vilib>:"WPI_RobotDriveDelayAndUpdateSafety.vi"("Delay (s)"=w196, "RobotDriveDevRef"=w201) -> ("RobotDriveDevRef 2"=w199:T4)  [unwired: 8 in, 1 out]
        n110 = call-poly <vilib>:"NT Write Value.vi"("Numeric Array"=w193, "Name"="RobotDrive Motors") -> ()  [unwired: 9 in, 1 out]
        "Current Movement, for debugging" <- w195
      }
    }
    frame "Alternative 2" {
      w203 = "RobotDrive Motors" ("Name")
      # "This is some simple sample code to drive your robot curving one direction and then the other."
      # "stand still"
      # "other way for 0.5 second"
      # "turn for 1 second"
      n111 = call <vilib>:"WPI_RobotDriveRefNum Registry Get.vi"("refnum name"="Left and Right Motors") -> ("RobotDriveDevRef"=w219:T4)  [unwired: 1 in, 9 out]
      n112 = call-poly <vilib>:"WPI_RobotDriveArcadeDrive.vi"("Y axis value"=0.5 ("X axis value"), "X axis value"=-0.25, "RobotDriveDevRef"=w219) -> ("Motor Values"=w202:dbl[], "RobotDriveDevRef"=w212:T4)  [unwired: 1 in, 6 out]
      n113 = call <vilib>:"WPI_RobotDriveDelayAndUpdateSafety.vi"("Delay (s)"=1.0, "RobotDriveDevRef"=w212) -> ("RobotDriveDevRef 2"=w213:T4)  [unwired: 8 in, 1 out]
      n114 = call-poly <vilib>:"WPI_RobotDriveArcadeDrive.vi"("Y axis value"=-0.25 ("X axis value"), "X axis value"=0.5, "RobotDriveDevRef"=w213) -> ("Motor Values"=w204:dbl[], "RobotDriveDevRef"=w214:T4)  [unwired: 1 in, 6 out]
      n115 = call <vilib>:"WPI_RobotDriveDelayAndUpdateSafety.vi"("Delay (s)"=0.5, "RobotDriveDevRef"=w214) -> ("RobotDriveDevRef 2"=w215:T4)  [unwired: 8 in, 1 out]
      n116 = call-poly <vilib>:"NT Write Value.vi"("Numeric Array"=w204, "Name"=w203) -> ()  [unwired: 9 in, 1 out]
      n117 = call-poly <vilib>:"NT Write Value.vi"("Numeric Array"=w202, "Name"=w203) -> ()  [unwired: 9 in, 1 out]
      n118 = call-poly <vilib>:"WPI_RobotDriveArcadeDrive.vi"("Y axis value"=0.0 ("X axis value"), "X axis value"=0.0, "RobotDriveDevRef"=w215) -> ("Motor Values"=w205:dbl[])  [unwired: 1 in, 7 out]
      n119 = call-poly <vilib>:"NT Write Value.vi"("Numeric Array"=w205, "Name"=w203) -> ()  [unwired: 9 in, 1 out]
    }
    frame Default {
      n120 = case shown="\"1\", Default" w220 {
        frame "2" {
          w222 = "RobotDrive Motors" ("Name")
          # "Straight for 3 seconds"
          n121 = call <vilib>:"WPI_RobotDriveRefNum Registry Get.vi"("refnum name"="Left and Right Motors") -> ("RobotDriveDevRef"=w238:T4)  [unwired: 1 in, 9 out]
          n122 = call-poly <vilib>:"WPI_RobotDriveArcadeDrive.vi"("Y axis value"=0.5 ("X axis value"), "X axis value"=0.0, "RobotDriveDevRef"=w238) -> ("Motor Values"=w226:dbl[], "RobotDriveDevRef"=w232:T4)  [unwired: 1 in, 6 out]
          n123 = call <vilib>:"WPI_RobotDriveDelayAndUpdateSafety.vi"("Delay (s)"=3.0, "RobotDriveDevRef"=w232) -> ("RobotDriveDevRef 2"=w233:T4)  [unwired: 8 in, 1 out]
          n124 = call-poly <vilib>:"WPI_RobotDriveArcadeDrive.vi"("Y axis value"=0.0 ("X axis value"), "X axis value"=0.5, "RobotDriveDevRef"=w233) -> ("Motor Values"=w227:dbl[], "RobotDriveDevRef"=w234:T4)  [unwired: 1 in, 6 out]
          n125 = call <vilib>:"WPI_RobotDriveDelayAndUpdateSafety.vi"("Delay (s)"=0.5, "RobotDriveDevRef"=w234) -> ("RobotDriveDevRef 2"=w221:T4)  [unwired: 8 in, 1 out]
          n126 = call-poly <vilib>:"NT Write Value.vi"("Numeric Array"=w227, "Name"=w222) -> ()  [unwired: 9 in, 1 out]
          n127 = call-poly <vilib>:"NT Write Value.vi"("Numeric Array"=w226, "Name"=w222) -> ()  [unwired: 9 in, 1 out]
          n128 = call-poly <vilib>:"WPI_RobotDriveArcadeDrive.vi"("Y axis value"=0.0 ("X axis value"), "X axis value"=0.0, "RobotDriveDevRef"=w221) -> ("Motor Values"=w223:dbl[])  [unwired: 1 in, 7 out]
          n129 = call-poly <vilib>:"NT Write Value.vi"("Numeric Array"=w223, "Name"=w222) -> ()  [unwired: 9 in, 1 out]
        }
        frame "3" {
          w261 = "RobotDrive Motors" ("Name")
          # "Straight for 3 seconds"
          n130 = call <vilib>:"WPI_RobotDriveRefNum Registry Get.vi"("refnum name"="Left and Right Motors") -> ("RobotDriveDevRef"=w239:T4)  [unwired: 1 in, 9 out]
          n131 = call-poly <vilib>:"WPI_RobotDriveArcadeDrive.vi"("Y axis value"=0.5 ("X axis value"), "X axis value"=0.0, "RobotDriveDevRef"=w239) -> ("Motor Values"=w255:dbl[], "RobotDriveDevRef"=w246:T4)  [unwired: 1 in, 6 out]
          n132 = call <vilib>:"WPI_RobotDriveDelayAndUpdateSafety.vi"("Delay (s)"=3.0, "RobotDriveDevRef"=w246) -> ("RobotDriveDevRef 2"=w245:T4)  [unwired: 8 in, 1 out]
          n133 = call-poly <vilib>:"WPI_RobotDriveArcadeDrive.vi"("Y axis value"=0.0 ("X axis value"), "X axis value"=-0.5, "RobotDriveDevRef"=w245) -> ("Motor Values"=w254:dbl[], "RobotDriveDevRef"=w244:T4)  [unwired: 1 in, 6 out]
          n134 = call <vilib>:"WPI_RobotDriveDelayAndUpdateSafety.vi"("Delay (s)"=0.5, "RobotDriveDevRef"=w244) -> ("RobotDriveDevRef 2"=w243:T4)  [unwired: 8 in, 1 out]
          n135 = call-poly <vilib>:"NT Write Value.vi"("Numeric Array"=w254, "Name"=w261) -> ()  [unwired: 9 in, 1 out]
          n136 = call-poly <vilib>:"NT Write Value.vi"("Numeric Array"=w255, "Name"=w261) -> ()  [unwired: 9 in, 1 out]
          n137 = call-poly <vilib>:"WPI_RobotDriveArcadeDrive.vi"("Y axis value"=0.5 ("X axis value"), "X axis value"=0.0, "RobotDriveDevRef"=w243) -> ("Motor Values"=w253:dbl[], "RobotDriveDevRef"=w259:T4)  [unwired: 1 in, 6 out]
          n138 = call <vilib>:"WPI_RobotDriveDelayAndUpdateSafety.vi"("Delay (s)"=0.5, "RobotDriveDevRef"=w259) -> ("RobotDriveDevRef 2"=w260:T4)  [unwired: 8 in, 1 out]
          n139 = call-poly <vilib>:"NT Write Value.vi"("Numeric Array"=w253, "Name"=w261) -> ()  [unwired: 9 in, 1 out]
          n140 = call-poly <vilib>:"WPI_RobotDriveArcadeDrive.vi"("Y axis value"=0.0 ("X axis value"), "X axis value"=0.0, "RobotDriveDevRef"=w260) -> ("Motor Values"=w262:dbl[])  [unwired: 1 in, 7 out]
          n141 = call-poly <vilib>:"NT Write Value.vi"("Numeric Array"=w262, "Name"=w261) -> ()  [unwired: 9 in, 1 out]
        }
        frame "1", Default {
          w278 = "RobotDrive Motors" ("Name")
          # "Step 6 Drive forward/put gear on hook"
          # "Step 5 Move forward/line up"
          # "Step 4 Turn 90 degrees to the left"
          # "Step 3 Drive Forward x feet"
          # "Step 2 Turn 90 degrees to the right"
          # "Step 1 Drive Forward for x feet"
          # "Stops Drive if Pressure\nSwitch is pressed"
          # "Stops Drive if Pressure\nSwitch is pressed"
          # "Stops Drive if Pressure\nSwitch is pressed"
          # "Straight for 3 seconds"
          n142 = call "Autonomous Encoder2 Read.vi"() -> ("error out"=w270:errorcluster, "Encoder Direction"=→"Encoder Direction":string, "Encoder Distance"=→"Encoder Distance":dbl)  [unwired: 9 in]
          n143 = call "Switch0 Pressed.vi"("error in (no error)"=w270) -> ("error out"=w272:errorcluster, "Switch Pressed"=w275:bool)  [unwired: 9 in]
          n144 = call <vilib>:"WPI_RobotDriveRefNum Registry Get.vi"("error in (no error)"=w272, "refnum name"="Left and Right Motors") -> ("RobotDriveDevRef"=w294:T4)  [unwired: 9 out]
          n145 = case shown="False" w275 {
            tunnel: w294 -> [w318 w326]
            tunnel: [w319 w325] -> w287
            tunnel: [w317 w323] -> w284
            tunnel: [w315 w321] -> w263
            frame False {
              n146 = call-poly <vilib>:"WPI_RobotDriveArcadeDrive.vi"("Y axis value"=-0.4 ("X axis value"), "X axis value"=0.0, "RobotDriveDevRef"=w318) -> ("error out"=w315:errorcluster, "Motor Values"=w317:dbl[], "RobotDriveDevRef"=w319:T4)  [unwired: 1 in, 5 out]
            }
            frame True {
              n147 = call-poly <vilib>:"WPI_RobotDriveArcadeDrive.vi"("Y axis value"=0.0 ("X axis value"), "X axis value"=0.0, "RobotDriveDevRef"=w326) -> ("error out"=w321:errorcluster, "Motor Values"=w323:dbl[], "RobotDriveDevRef"=w325:T4)  [unwired: 1 in, 5 out]
            }
          }
          "Motor Values" <- w284
          n148 = call "Autonomous Encoder2 Read.vi"("error in (no error)"=w263) -> ("error out"=w265:errorcluster, "Encoder Direction"=→"Encoder Direction 2":string, "Encoder Distance"=→"Encoder Distance 2":dbl)  [unwired: 8 in]
          n149 = call "Switch0 Pressed.vi"("error in (no error)"=w265) -> ("error out"=w264:errorcluster, "Switch Pressed"=w274:bool)  [unwired: 9 in]
          n150 = call <vilib>:"WPI_RobotDriveDelayAndUpdateSafety.vi"("error in (no error)"=w264, "Delay (s)"=5.0, "RobotDriveDevRef"=w287) -> ("RobotDriveDevRef 2"=w288:T4)  [unwired: 7 in, 1 out]
          n151 = call "Switch0 Pressed.vi"() -> ("Switch Pressed"=→"Switch Pressed":bool)  [unwired: 10 in, 1 out]
          n152 = case shown="False" w274 {
            tunnel: [w307 w314] -> w289
            tunnel: w288 -> [w306 w313]
            tunnel: [w305 w310] -> w285
            frame False {
              n153 = call-poly <vilib>:"WPI_RobotDriveArcadeDrive.vi"("Y axis value"=0.4 ("X axis value"), "X axis value"=0.0, "RobotDriveDevRef"=w306) -> ("Motor Values"=w305:dbl[], "RobotDriveDevRef"=w307:T4)  [unwired: 1 in, 6 out]
            }
            frame True {
              n154 = call-poly <vilib>:"WPI_RobotDriveArcadeDrive.vi"("Y axis value"=0.0 ("X axis value"), "X axis value"=0.0, "RobotDriveDevRef"=w313) -> ("Motor Values"=w310:dbl[], "RobotDriveDevRef"=w314:T4)  [unwired: 1 in, 6 out]
            }
          }
          n155 = call <vilib>:"WPI_RobotDriveDelayAndUpdateSafety.vi"("Delay (s)"=3.0, "RobotDriveDevRef"=w289) -> ("error out"=w271:errorcluster, "RobotDriveDevRef 2"=w290:T4)  [unwired: 8 in]
          n156 = call-poly <vilib>:"NT Write Value.vi"("Numeric Array"=w285, "Name"=w278) -> ()  [unwired: 9 in, 1 out]
          n157 = call-poly <vilib>:"NT Write Value.vi"("Numeric Array"=w284, "Name"=w278) -> ()  [unwired: 9 in, 1 out]
          n158 = call "Switch0 Pressed.vi"("error in (no error)"=w271) -> ("Switch Pressed"=w273:bool)  [unwired: 9 in, 1 out]
          n159 = case shown="False" w273 {
            tunnel: w290 -> [w297 w304]
            tunnel: [w295 w301] -> w286
            tunnel: [w296 w300] -> w280
            frame False {
              n160 = call-poly <vilib>:"WPI_RobotDriveArcadeDrive.vi"("Y axis value"=0.0 ("X axis value"), "X axis value"=-0.4, "RobotDriveDevRef"=w297) -> ("Motor Values"=w295:dbl[], "RobotDriveDevRef"=w296:T4)  [unwired: 1 in, 6 out]
            }
            frame True {
              n161 = call-poly <vilib>:"WPI_RobotDriveArcadeDrive.vi"("Y axis value"=0.0 ("X axis value"), "X axis value"=0.0, "RobotDriveDevRef"=w304) -> ("Motor Values"=w301:dbl[], "RobotDriveDevRef"=w300:T4)  [unwired: 1 in, 6 out]
            }
          }
          n162 = call <vilib>:"WPI_RobotDriveDelayAndUpdateSafety.vi"("Delay (s)"=0.5, "RobotDriveDevRef"=w280) -> ("RobotDriveDevRef 2"=w279:T4)  [unwired: 8 in, 1 out]
          n163 = call-poly <vilib>:"NT Write Value.vi"("Numeric Array"=w286, "Name"=w278) -> ()  [unwired: 9 in, 1 out]
          n164 = call-poly <vilib>:"WPI_RobotDriveArcadeDrive.vi"("Y axis value"=0.0 ("X axis value"), "X axis value"=0.0, "RobotDriveDevRef"=w279) -> ("Motor Values"=w277:dbl[])  [unwired: 1 in, 7 out]
          n165 = call-poly <vilib>:"NT Write Value.vi"("Numeric Array"=w277, "Name"=w278) -> ()  [unwired: 9 in, 1 out]
        }
      }
    }
  }
  n166 = Index Array(array=w3, index #1=2 ("index")) -> ()  [unwired: 1 in, 2 out]
  n167 = call-poly <vilib>:"NT Write Value.vi"("Numeric Array"=w3, "Name"="Joystick 0/Axes") -> ()  [unwired: 9 in, 1 out]
  n168 = disable-structure shown="Enabled" {
    frame Disabled {
      w340 = FPGA_DIOChannel."DIO 1"  # B Channel
      w339 = FPGA_DIOChannel."DIO 0"  # A Channel
      # "in inches"
      n169 = call <vilib>:"WPI_DigitalInputOpen.vi"("DIO Channel"=w339) -> ("DigitalInputDevRef"=w336:T10)  [unwired: 1 in, 9 out]
      n170 = call <vilib>:"WPI_DigitalInputOpen.vi"("DIO Channel"=w340) -> ("DigitalInputDevRef"=w337:T10)  [unwired: 1 in, 9 out]
      n171 = call-poly <vilib>:"WPI_CounterToDigitalSource.vi"("DigitalInputDevRef"=w336) -> ("Digital Source"=w335:T11)  [unwired: 6 out]
      n172 = call-poly <vilib>:"WPI_CounterToDigitalSource.vi"("DigitalInputDevRef"=w337) -> ("Digital Source"=w338:T11)  [unwired: 6 out]
      n173 = call <vilib>:"WPI_EncoderOpen.vi"("DistancePerCount"=18.84955592153876, "Invert Direction (False)"=FALSE, "BSource"=w338, "ASource"=w335) -> ("error out"=w333:errorcluster, "EncoderDevRef"=w334:T15)  [unwired: 4 in, 2 out]
      n174 = call <vilib>:"WPI_EncoderRefNum Registry Set.vi"("error in (no error)"=w333, "refnum name"="Encoder", "EncoderDevRef"=w334) -> ("error out"=w331:errorcluster, "EncoderDevRef"=w332:T15)  [unwired: 7 in]
      n175 = call <vilib>:"WPI_EncoderGet.vi"("error in (no error)"=w331, "EncoderDevRef"=w332) -> ()  [unwired: 4 in, 6 out]
      n176 = call-poly <vilib>:"NT Write Value.vi"("Name"="Encoder Distance") -> ()  [unwired: 10 in, 1 out]
    }
    frame Enabled {
    }
  }
